vi "MC Read ADC Channel.vi"(1 "Range (+/- 10V)":i32(ring) items=["Not Programmable", "+- 10 V", "+- 5 V", "+- 2.5 V", "+- 1.67 V", "+- 1.25 V", "+- 1 V", "+- .625 V", "+- .5 V", "+- .1 V", "+- .05 V", "+- .01 V", "+- .005 V", "0 - 10 V", "0 - 5 V", "0 - 2.5 V", "0 - 2 V", "0 - 1.67 V", "0 - 1.25 V", "0 - 1 V", "0 - .1 V", "0 - .01 V", "4-20 mA", "2-10 mA", "1-5 mA", "0.5-2.5 mA"], 2 "Channel (0)":i32, 3 "BoardNum (0)":u32) -> (0 "Output":sgl format="%.5f")   [LabVIEW 2010]
uses:
  <vilib>/ULx/Create Channel.llb/ULx Create Channel (AI-Current-Basic).vi
  <vilib>/ULx/Create Channel.llb/ULx Create Channel (AI-Voltage-Basic).vi
  <vilib>/ULx/Timing.llb/ULx Timing (Sample Clock).vi
  <vilib>/ULx/Read.llb/ULx Read (Analog 1D DBL 1Chan NSamp).vi
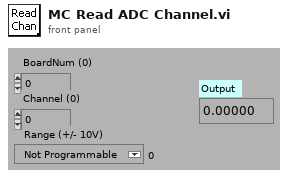
[diagram p1: front panel]
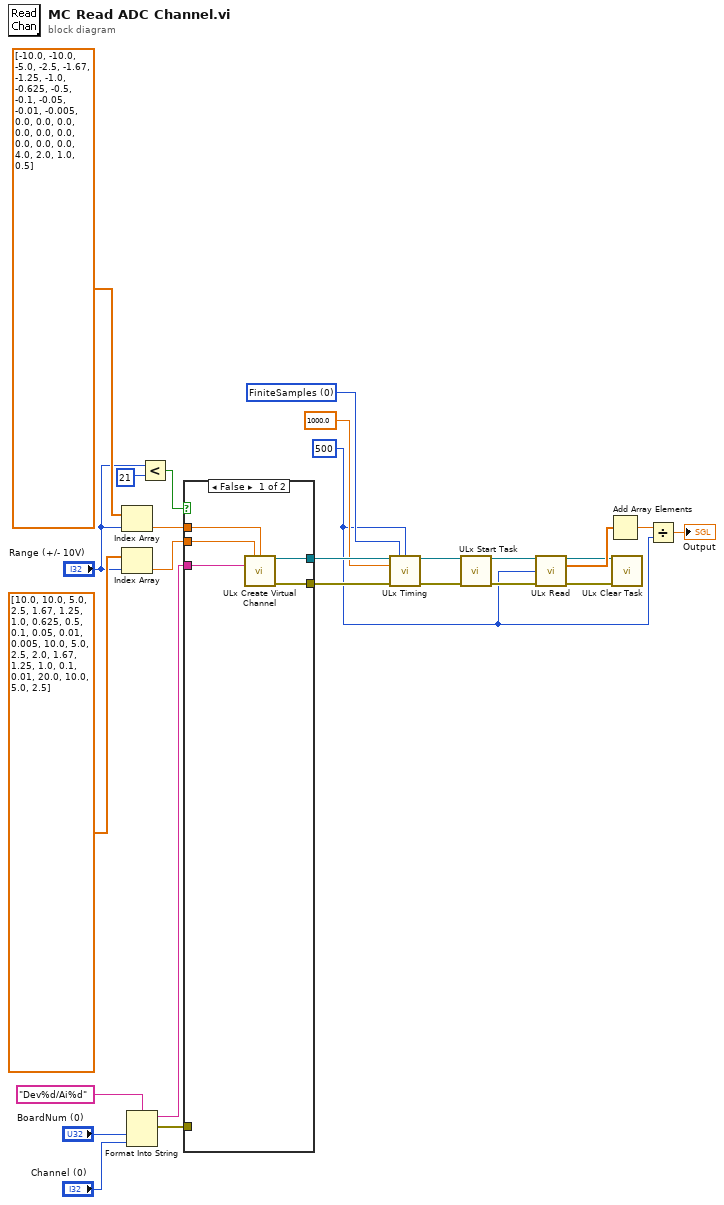
[diagram p0: block diagram]
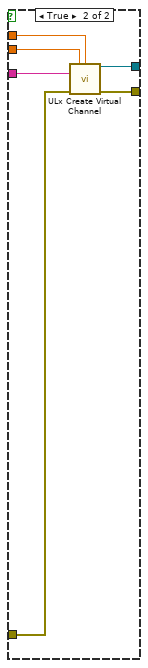
[diagram p2: hidden frame]
diagram:
  w9 = 0 items=["FiniteSamples", "ContinuousSamples"] ("sample mode")
  w8 = 500 ("number of samples per channel")
  n1 = Index Array(array=dbl[] [-10.0, -10.0, -5.0, -2.5, -1.67, -1.25, -1.0, -0.625, -0.5, -0.1, -0.05, -0.01, -0.005, 0.0, 0.0, 0.0, 0.0, 0.0, 0.0, 0.0, 0.0, 0.0, 4.0, 2.0, 1.0, 0.5], index="Range (+/- 10V)") -> (element=w24:dbl)
  n2 = Index Array(array=dbl[] [10.0, 10.0, 5.0, 2.5, 1.67, 1.25, 1.0, 0.625, 0.5, 0.1, 0.05, 0.01, 0.005, 10.0, 5.0, 2.5, 2.0, 1.67, 1.25, 1.0, 0.1, 0.01, 20.0, 10.0, 5.0, 2.5], index="Range (+/- 10V)") -> (element=w23:dbl)
  n3 = Format Into String(format string="Dev%d/Ai%d", "BoardNum (0)", "Channel (0)") -> (resulting string=w1:string, error out=w2:errorcluster)  [unwired: 2 in]
  n4 = Less?(x="Range (+/- 10V)", y=21) -> (x < y?=w20:bool)
  n5 = case shown="False" w20 {
    tunnel: w24 -> [w30 w37]
    tunnel: w23 -> [w31 w36]
    tunnel: [w29 w35] -> w14
    tunnel: [w28 w34] -> w13
    tunnel: w2 -> [_ w33]
    tunnel: w1 -> [w27 w32]
    frame False {
      n6 = call-poly <vilib>:"ULx Create Virtual Channel.vi"("maximum value"=w31, "minimum value"=w30, "physical channels"=w27) -> ("task out"=w29:refnum<k24>, "error out"=w28:errorcluster)  [unwired: 11 in]
    }
    frame True {
      n7 = call-poly <vilib>:"ULx Create Virtual Channel.vi"("maximum value"=w36, "minimum value"=w37, "physical channels"=w32, "error in"=w33) -> ("task out"=w35:refnum<k24>, "error out"=w34:errorcluster)  [unwired: 10 in]
    }
  }
  n8 = call-poly <vilib>:"ULx Timing.vi"("task in"=w14, "sample mode"=w9, "samples per channel"=w8, "rate"=1000.0, "error in"=w13) -> ("task out"=w12:refnum<k24>, "error out"=w11:errorcluster)  [unwired: 9 in]
  n9 = call <vilib>:"ULx Start Task.vi"("task in"=w12, "error in"=w11) -> ("task out"=w19:refnum<k24>, "error out"=w18:errorcluster)  [unwired: 12 in]
  n10 = call-poly <vilib>:"ULx Read.vi"("task in"=w19, "number of samples per channel"=w8, "error in"=w18) -> ("task out"=w6:refnum<k24>, "data"=w17:dbl[], "error out"=w7:errorcluster)  [unwired: 10 in]
  n11 = Add Array Elements(numeric array=w17) -> (sum=w16:dbl)
  n12 = call <vilib>:"ULx Clear Task.vi"("task in"=w6, "error in"=w7) -> ()  [unwired: 13 in, 1 out]
  n13 = Divide(x=w16, y=w8) -> (x/y=→"Output":dbl)
